vi "readTag.vi"(8 "error in (no error)":errorcluster, 11 "ESP8266 in":refnum<class "ESP8266.lvclass">) -> (0 "error out":errorcluster, 3 "ESP8266 out":refnum<class "ESP8266.lvclass">)   [LabVIEW 2020, in "ESP8266.lvclass"]
uses:
  ESP8266.lvclass
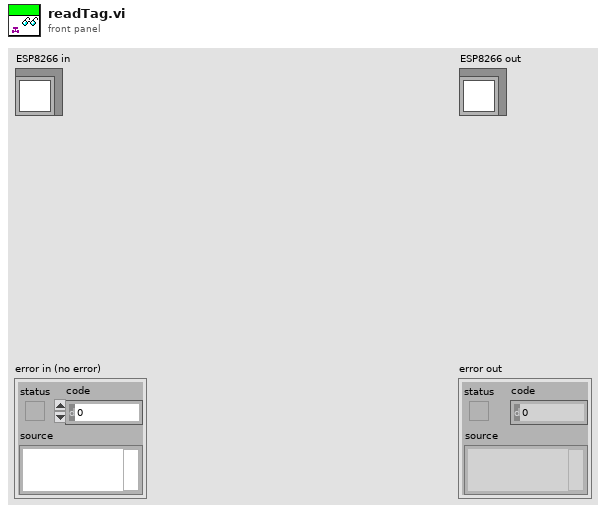
[diagram p1: front panel]
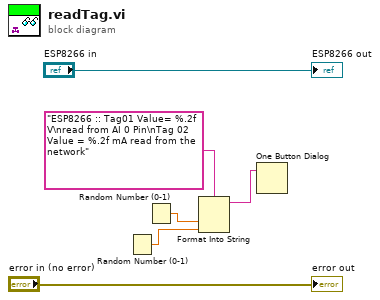
[diagram p0: block diagram]
diagram:
  n1 = Random Number (0-1)() -> (number: 0 to 1=w1:dbl)
  n2 = Random Number (0-1)() -> (number: 0 to 1=w3:dbl)
  n3 = Format Into String(format string="ESP8266 :: Tag01 Value= %.2f V\nread from AI 0 Pin\nTag 02 Value = %.2f mA read from the network" ("message"), w3, w1) -> (resulting string=w2:string)  [unwired: 2 in, 1 out]
  n4 = One Button Dialog(message=w2) -> ()  [unwired: 1 in, 1 out]
  "error out" <- "error in (no error)"
  "ESP8266 out" <- "ESP8266 in"
